vi "Mappa AO PLC_2.vi"(11 "USCITE PLC 2":T1={"AO (real) 2"={"SCORTA 1"=0.0, "SCORTA 2"=0.0, "SCORTA 3"=0.0, "SCORTA 4"=0.0, "SCORTA 5"=0.0, "SCORTA 6"=0.0, "SCORTA 7"=0.0, "SCORTA 8"=0.0}, "statoAO_PLC out"={"Condensatori"=nan, "Scorta 1"=nan, "Scorta 2"=0.0}, "DO (bit)"={"Relè misura resistomat"=FALSE, "Misura res ramo 1"=FALSE, "Misura res ramo 2"=FALSE, "Misura res ramo 3"=FALSE, "Scelta banco 2"=FALSE, "Scala Torsiometro"=FALSE, "Ctrl torsiometro"=FALSE, "Select current mode"=FALSE, "Select Torque mode"=FALSE, "Select speed mode"=FALSE, "Watchdog"=FALSE, "Scorta"=FALSE, "Scorta 2"=FALSE, "Scorta 3"=FALSE, "Scorta 4"=FALSE, "Scorta 5"=FALSE, "Bench selection"=FALSE, "External alarm"=FALSE, "Enable external program"=FALSE, "Reset allarmi"=FALSE, "Start"=FALSE, "Stop"=FALSE, "Block"=FALSE, "Scorta 6"=FALSE}}) -> (0 "Array DB REAL out":dbl[](array[numeric]), 1 "Array DB W out":dbl[](array[numeric]), 2 "Array M REAL out":dbl[](array[numeric]), 3 "Array M WORD out":dbl[](array[numeric]))   [LabVIEW 2019]
uses:
  Uscite PLC 2.ctl
  controls/statoAO_plc_2.ctl
  StatoDO_PLC_2.ctl
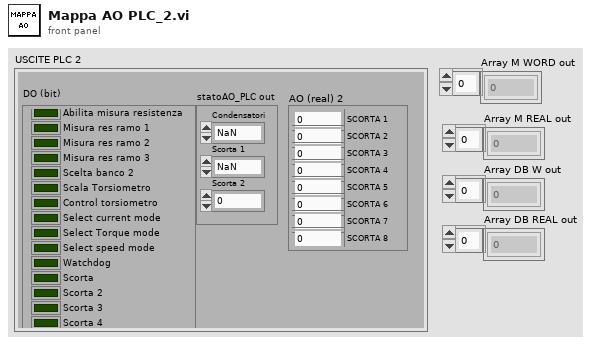
[diagram p1: front panel]
types:
  T1 = typedef "Uscite PLC 2.ctl" = cluster{"AO (real) 2":cluster{"SCORTA 1":dbl, "SCORTA 2":dbl, "SCORTA 3":dbl, "SCORTA 4":dbl, "SCORTA 5":dbl, "SCORTA 6":dbl, "SCORTA 7":dbl, "SCORTA 8":dbl}, "statoAO_PLC out":T2, "DO (bit)":T3}
  T2 = typedef "statoAO_plc_2.ctl" = cluster{"Condensatori":dbl, "Scorta 1":dbl, "Scorta 2":dbl}
  T3 = typedef "StatoDO_PLC_2.ctl" = cluster{"Relè misura resistomat":bool, "Misura res ramo 1":bool, "Misura res ramo 2":bool, "Misura res ramo 3":bool, "Scelta banco 2":bool, "Scala Torsiometro":bool, "Ctrl torsiometro":bool, "Select current mode":bool, "Select Torque mode":bool, "Select speed mode":bool, "Watchdog":bool, "Scorta":bool, "Scorta 2":bool, "Scorta 3":bool, "Scorta 4":bool, "Scorta 5":bool, "Bench selection":bool, "External alarm":bool, "Enable external program":bool, "Reset allarmi":bool, "Start":bool, "Stop":bool, "Block":bool, "Scorta 6":bool}
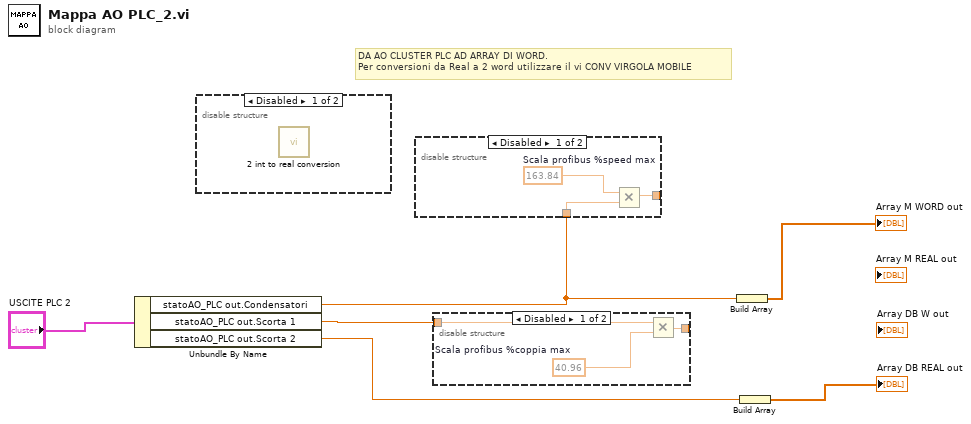
[diagram p0: block diagram]
diagram:
  # "DA AO CLUSTER PLC AD ARRAY DI WORD.\nPer conversioni da Real a 2 word utilizzare il vi CONV VIRGOLA MOBILE"
  n1 = Unbundle By Name("USCITE PLC 2") -> ("statoAO_PLC out.Condensatori"=w2:dbl, "statoAO_PLC out.Scorta 1"=w5:dbl, "statoAO_PLC out.Scorta 2"=w4:dbl)
  n2 = disable-structure shown="Disabled" {
    frame Disabled {
      n3 = call "2 int to real conversion.vi"() -> ()  [unwired: 9 in, 3 out]
    }
    frame Enabled {
    }
  }
  n4 = disable-structure shown="Disabled" {
    disable-tunnel: w2 -> [w9 _]
    disable-tunnel: [w8 _] -> _
    frame Disabled {
      w7 = 163.84  # Scala profibus %speed max
      n5 = Multiply(x=w7, y=w9) -> (x*y=w8:dbl)
    }
    frame Enabled {
    }
  }
  n6 = disable-structure shown="Disabled" {
    disable-tunnel: w5 -> [w12 _]
    disable-tunnel: [w11 _] -> _
    frame Disabled {
      w10 = 40.96  # Scala profibus %coppia max
      n7 = Multiply(x=w12, y=w10) -> (x*y=w11:dbl)
    }
    frame Enabled {
    }
  }
  n8 = Build Array(w2) -> (→"Array M WORD out":dbl[])
  n9 = Build Array(w4) -> (→"Array DB REAL out":dbl[])
